vi "Parse Boolean Array.vi"(8 "error in (no error)":errorcluster, 11 "Bool Array Input":bool[](array[boolean])) -> (0 "error out":errorcluster, 3 "output cluster":T1)   [LabVIEW 2018]
uses:
  Ctls/DisplayIndicator.ctl
  Ctls/MotroConfigData.ctl
  Ctls/MotorConfig.ctl
  Ctls/MagType.ctl
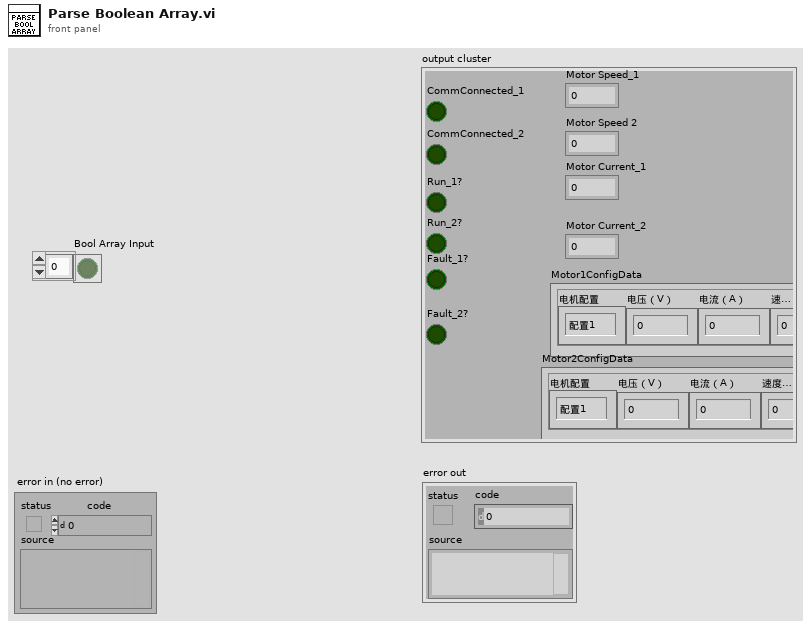
[diagram p1: front panel]
types:
  T1 = typedef "DisplayIndicator.ctl" = cluster{"CommConnected_1":bool, "Run_1?":bool, "Fault_1?":bool, "CommConnected_2":bool, "Run_2?":bool, "Fault_2?":bool, "Motor Speed 2":sgl, "Motor Speed_1":sgl, "Motor Current_1":sgl, "Motor Current_2":sgl, "Motor1ConfigData":T2, "Motor2ConfigData":T2}
  T2 = typedef "MotroConfigData.ctl" = cluster{"电机配置":T3, "电压（V）":dbl, "电流（A）":dbl, "速度（RPM）":dbl, "励磁方式":T4}
  T3 = typedef "MotorConfig.ctl" = enum16{"配置1", "配置2", "配置3", "配置4"}
  T4 = typedef "MagType.ctl" = enum16{"永磁", "励磁"}
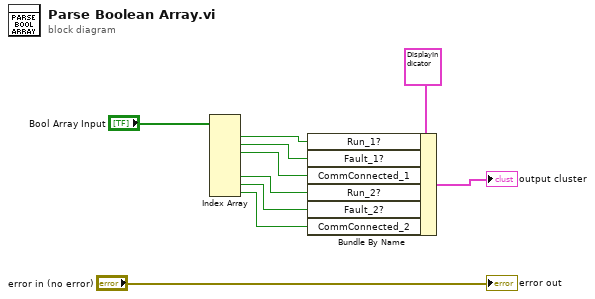
[diagram p0: block diagram]
diagram:
  n1 = Index Array(array="Bool Array Input") -> (element #1=w9:bool, element #2=w8:bool, element #3=w7:bool, element #6=w6:bool, element #7=w5:bool, element #8=w4:bool)  [unwired: 8 in, 2 out]
  n2 = Bundle By Name(cluster=T1 {"CommConnected_1"=FALSE, "Run_1?"=FALSE, "Fault_1?"=FALSE, "CommConnected_2"=FALSE, "Run_2?"=FALSE, "Fault_2?"=FALSE, "Motor Speed 2"=0.0, "Motor Speed_1"=0.0, "Motor Current_1"=0.0, "Motor Current_2"=0.0, "Motor1ConfigData"={"电机配置"=enum."配置1", "电压（V）"=0.0, "电流（A）"=0.0, "速度（RPM）"=0.0, "励磁方式"=enum."永磁"}, "Motor2ConfigData"={"电机配置"=enum."配置1", "电压（V）"=0.0, "电流（A）"=0.0, "速度（RPM）"=0.0, "励磁方式"=enum."永磁"}} ("Display"), "Run_1?"=w9, "Fault_1?"=w8, "CommConnected_1"=w7, "Run_2?"=w6, "Fault_2?"=w5, "CommConnected_2"=w4) -> (→"output cluster":T1)
  "error out" <- "error in (no error)"
